vi "Read_queueTcpClientFromDdsMaxSize.vi"(8 "error in (no error)":errorcluster, 11 "TcpServerTel in":refnum<class "TcpServerTel.lvclass">) -> (0 "error out":errorcluster, 2 "queueTcpClientFromDdsMaxSize":i32=1000, 3 "TcpServerTel out":refnum<class "TcpServerTel.lvclass">)   [LabVIEW 2018, in "TcpServerTel.lvclass"]
doc: "Read the queueTcpClientFromDdsMaxSize."
uses:
  TcpServerTel.lvclass
  TcpServerTel.lvclass/TcpServerTel.ctl
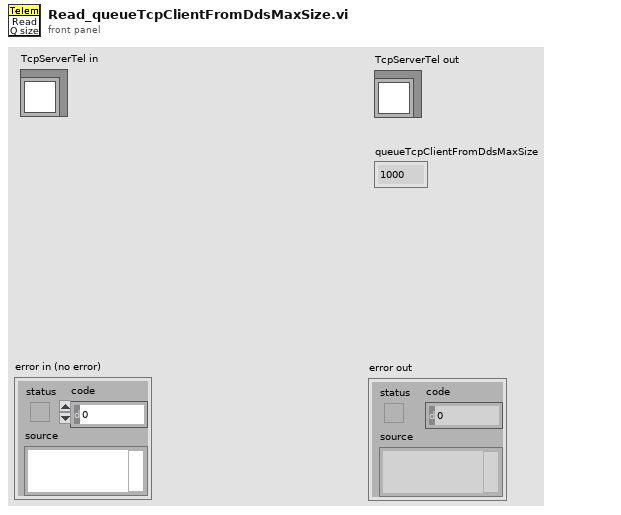
[diagram p1: front panel]
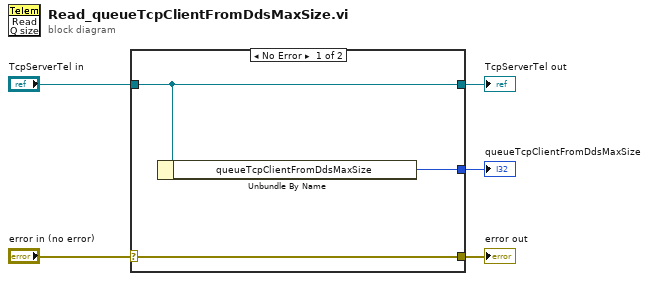
[diagram p0: block diagram]
diagram:
  n1 = case shown="No Error" "error in (no error)" {
    selector: "error in (no error)" -> [w8 w9]
    tunnel: [w8 w9] -> w4
    tunnel: [w7 w10] -> w2
    tunnel: "TcpServerTel in" -> [w7 w10]
    tunnel: [w6 _] -> w1
    frame No Error {
      n2 = Unbundle By Name(w7) -> ("queueTcpClientFromDdsMaxSize"=w6:i32)
    }
    frame Error {
    }
  }
  "error out" <- w4
  "TcpServerTel out" <- w2
  "queueTcpClientFromDdsMaxSize" <- w1
